vi "Telescope Close.vi"(8 "error in (no error)":errorcluster, 11 "LDT Telescope in":refnum<class "LDT Telescope.lvclass">) -> (0 "error out":errorcluster, 3 "LDT Telescope out":refnum<class "LDT Telescope.lvclass">)   [LabVIEW 2022 SP3, in "LDT Telescope.lvclass"]
uses:
  LDT Telescope.lvclass
  LDT Telescope.lvclass/LDT Telescope.ctl
  Telescope.lvclass
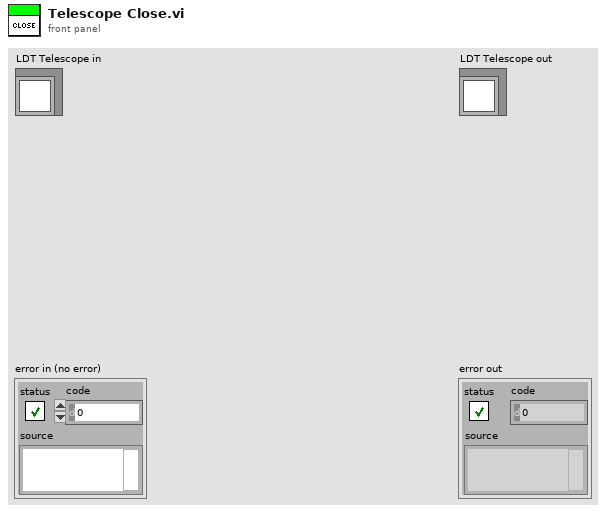
[diagram p1: front panel]
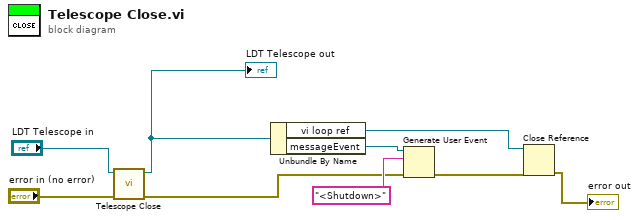
[diagram p0: block diagram]
diagram:
  n1 = call-parent "Telescope Close.vi"("error in (no error)"="error in (no error)", "Telescope in"="LDT Telescope in") -> ("error out"=w4:errorcluster, "Telescope out"=w7:refnum<class "LDT Telescope.lvclass">)  [unwired: 8 in]
  "LDT Telescope out" <- w7
  n2 = Unbundle By Name(w7) -> ("vi loop ref"=w3:refnum<vi>, "messageEvent"=w6:refnum<user-event>)
  n3 = Generate User Event(user event=w6, event data cluster="<Shutdown>" ("event data"), error in=w4) -> (error out=w2:errorcluster)  [unwired: 1 in, 1 out]
  n4 = Close Reference(reference=w3, error in (no error)=w2) -> (error out=→"error out":errorcluster)
